vi "Close.vi"(8 "error in (no error)":errorcluster, 10 "Msg in":T1, 11 "FakePressureController in":refnum<class "DaqPad_NI6009.lvclass">) -> (0 "error out":errorcluster, 1 "new command":string, 2 "Msg out":T1, 3 "FakePressureController out":refnum<class "DaqPad_NI6009.lvclass">)   [LabVIEW 2011, in "DaqPad_NI6009.lvclass"]
uses:
  DaqPad_NI6009.lvclass
  DriverMsg.ctl
  BaseDriver/BaseDriver.lvclass
  DaqPad_NI6009.lvclass/DaqPad_NI6009.ctl
  DAQmx Fill In Error Info.vi
  C:/Program Files/National Instruments/LabVIEW 2011/resource/objmgr/daqmx.rc
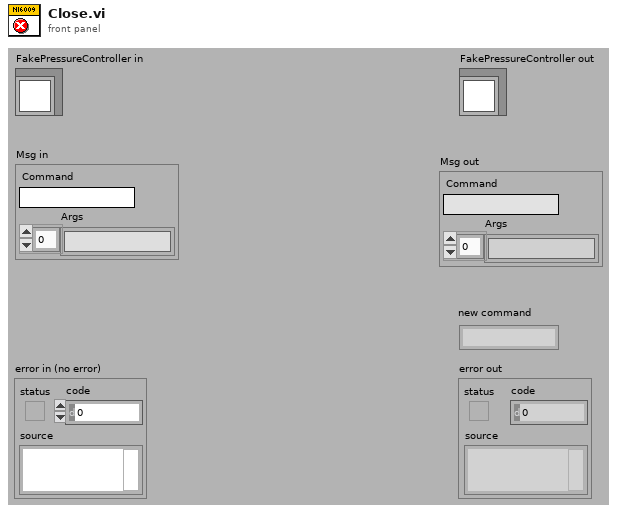
[diagram p1: front panel]
types:
  T1 = typedef "DriverMsg.ctl" = cluster{"Command":string, "Args":string[]}
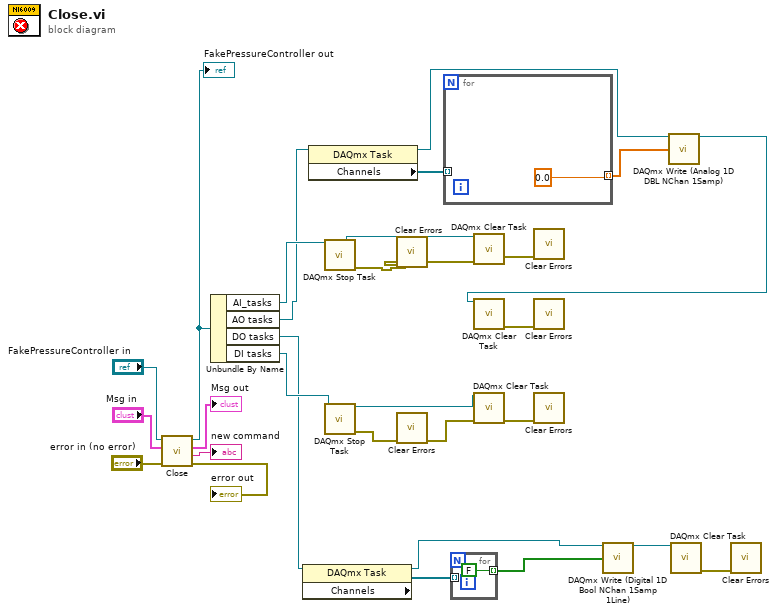
[diagram p0: block diagram]
diagram:
  n1 = call-parent "Close.vi"("error in (no error)"="error in (no error)", "Msg in"="Msg in", "BaseDriver in"="FakePressureController in") -> ("error out"=→"error out":errorcluster, "new command"=→"new command":string, "Msg out"=→"Msg out":T1, "BaseDriver out"=w24:refnum<class "DaqPad_NI6009.lvclass">)  [unwired: 5 in]
  "FakePressureController out" <- w24
  n2 = Unbundle By Name(w24) -> ("AI_tasks"=w11:refnum<k21>, "AO tasks"=w10:refnum<k21>, "DO tasks"=w5:refnum<k21>, "DI tasks"=w17:refnum<k21>)
  n3 = property class="DAQmx Task"(reference=w5) -> (reference out=w4:refnum<k21>, "Channels"=w6:refnum<k21>[])  [unwired: 1 in, 1 out]
  n4 = property class="DAQmx Task"(reference=w10) -> (reference out=w7:refnum<k21>, "Channels"=w9:refnum<k21>[])  [unwired: 1 in, 1 out]
  n5 = call "DAQmx Stop Task.vi"("task/channels in"=w11) -> ("task out"=w18:refnum<k21>, "error out"=w15:errorcluster)  [unwired: 13 in]
  n6 = call "DAQmx Stop Task.vi"("task/channels in"=w17) -> ("task out"=w16:refnum<k21>, "error out"=w13:errorcluster)  [unwired: 13 in]
  n7 = call "Clear Errors.vi"("error in (no error)"=w15) -> ("error out"=w14:errorcluster)  [unwired: 6 in]
  n8 = call "Clear Errors.vi"("error in (no error)"=w13) -> ("error out"=w12:errorcluster)  [unwired: 6 in]
  n9 = for {
    tunnel: w9 -> [_] mode=indexing
    tunnel: [0.0] -> w8 mode=indexing
  }
  n10 = for {
    tunnel: w6 -> [_] mode=indexing
    tunnel: [FALSE] -> w3 mode=indexing
  }
  n11 = call "DAQmx Clear Task.vi"("task in"=w18, "error in"=w14) -> ("error out"=w23:errorcluster)  [unwired: 13 in]
  n12 = call "DAQmx Clear Task.vi"("task in"=w16, "error in"=w12) -> ("error out"=w19:errorcluster)  [unwired: 13 in]
  n13 = call "Clear Errors.vi"("error in (no error)"=w23) -> ()  [unwired: 6 in, 1 out]
  n14 = call "Clear Errors.vi"("error in (no error)"=w19) -> ()  [unwired: 6 in, 1 out]
  n15 = call "DAQmx Write (Digital 1D Bool NChan 1Samp 1Line).vi"("task/channels in"=w4, "data"=w3) -> ("task out"=w2:refnum<k21>)  [unwired: 11 in, 2 out]
  n16 = call "DAQmx Write (Analog 1D DBL NChan 1Samp).vi"("task/channels in"=w7, "data"=w8) -> ("task out"=w1:refnum<k21>)  [unwired: 11 in, 2 out]
  n17 = call "DAQmx Clear Task.vi"("task in"=w1) -> ("error out"=w21:errorcluster)  [unwired: 14 in]
  n18 = call "Clear Errors.vi"("error in (no error)"=w21) -> ()  [unwired: 6 in, 1 out]
  n19 = call "DAQmx Clear Task.vi"("task in"=w2) -> ("error out"=w20:errorcluster)  [unwired: 14 in]
  n20 = call "Clear Errors.vi"("error in (no error)"=w20) -> ()  [unwired: 6 in, 1 out]
